vi "ClusterInfo.vi"() -> ()   [LabVIEW 2011]
uses:
  source_dilution.ctl
  source_noDilution.ctl
panel:
  in  "Al bubbler":T1 caption="Al" {"Flow" format="%.2f"}
  out "Array 2":string[](array[string])
  out "Array":u32[](array[numeric])
  out "size(s)":i32
  in  "Ga bubbler":T2={"Dilution"=FALSE, "Calculated"=0, "MFC1 flow"=0.0, "MFC2 flow"=10.0, "MFC3 flow"=100.0, "Main"={"Flow"=0.0, "Prep"=FALSE, "Run"=FALSE, "Active"=FALSE, "Name"=""}} caption="Al" {"Main"."Flow" format="%.2f"; "MFC1 flow" format="%.4f"; "MFC3 flow" format="%.1f"; "MFC2 flow" format="%.2f"; "Calculated" items=["Flow", "MFC1", "MFC2", "MFC3"]}
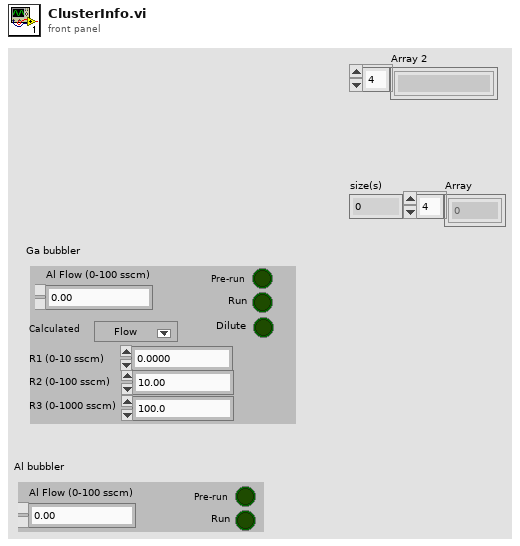
[diagram p1: front panel]
types:
  T1 = typedef "source_noDilution.ctl" = cluster{"Flow":dbl, "Prep":bool, "Run":bool, "Active":bool, "Name":string}
  T2 = typedef "source_dilution.ctl" = cluster{"Dilution":bool, "Calculated":u16, "MFC1 flow":dbl, "MFC2 flow":dbl, "MFC3 flow":dbl, "Main":T1}
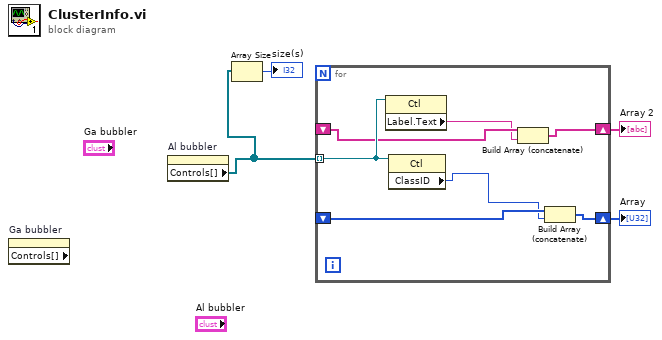
[diagram p0: block diagram]
diagram:
  n1 = property on="Ga bubbler" class="Clust (strict)" props=["Controls[]"]() -> ()  [unwired: 2 in, 3 out]
  n2 = property on="Al bubbler" class="Clust (strict)"() -> ("Controls[]"=w1:refnum<vi>[])  [unwired: 2 in, 2 out]
  n3 = Array Size(array=w1) -> (size(s)=→"size(s)":i32)
  n4 = for {
    tunnel: w1 -> [w10] mode=indexing
    shift-right: [w11] -> w3
    shift-left: _ -> [w6]
    shift-right: [w9] -> w2
    shift-left: _ -> [w8]
    n5 = property class="Ctl"(reference=w10) -> ("Label.Text"=w7:string)  [unwired: 1 in, 2 out]
    n6 = property class="Ctl"(reference=w10) -> ("ClassID"=w5:u32)  [unwired: 1 in, 2 out]
    n7 = Build Array (concatenate)(w8, w7) -> (w9:string[])
    n8 = Build Array (concatenate)(w6, w5) -> (w11:u32[])
  }
  "Array" <- w3
  "Array 2" <- w2
